vi "Inst_Initial.vi"(9 "error in (no error)":errorcluster, 10 "Combo Box":string(combo), 11 "VISA resource name 4":refnum<visa-resource-name>="FT6301A") -> (1 "error out":errorcluster, 3 "instrument ok?":bool)   [LabVIEW 2023]
panel:
  out "read buffer":string
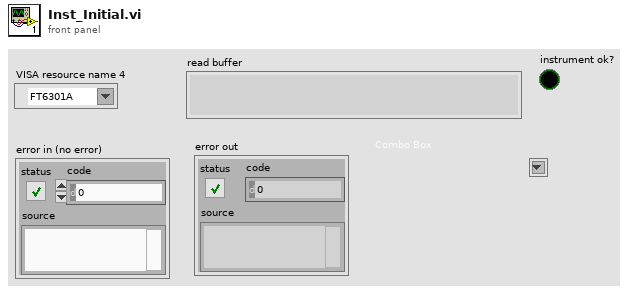
[diagram p1: front panel]
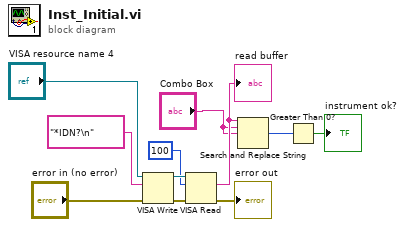
[diagram p0: block diagram]
diagram:
  n1 = VISA Write(VISA resource name="VISA resource name 4", write buffer="*IDN?\n", error in (no error)="error in (no error)") -> (VISA resource name out=w9:refnum<visa-resource-name>, error out=w8:errorcluster)  [unwired: 1 out]
  n2 = VISA Read(VISA resource name=w9, byte count=u32 100, error in (no error)=w8) -> (read buffer=w6:string, error out=→"error out":errorcluster)  [unwired: 2 out]
  "read buffer" <- w6
  n3 = Search and Replace String(input string=w6, search string="Combo Box", replace string="Combo Box") -> (number of replacements=w5:i32)  [unwired: 5 in, 3 out]
  n4 = Greater Than 0?(x=w5) -> (x > 0?=→"instrument ok?":bool)
